vi "rsp_Show Worker Front Panel.vi"(4 "Show in Debugger?":bool=TRUE, 6 "Message Priority":T1=enum."Normal", 8 "error in":errorcluster, 9 "Data in":T2, 11 "Application Manager in":refnum<class "Application Manager.lvclass">) -> (0 "error out":errorcluster, 3 "dup Application Manager out":refnum<class "Application Manager.lvclass">)   [LabVIEW 2017, in "Application Manager.lvclass"]
doc: "This VI sends a <b>Public API Response</b> message to a registered MHL case of the Caller of the Worker that owns this VI.\n---"
uses:
  Application Manager.lvclass
  C:/Program Files (x86)/National Instruments/LabVIEW 2017/vi.lib/addons/_Workers/Library/Classes/Worker/Worker.lvclass
  rsp_Show Worker Front Panel.ctl
  Common VIs/DC_UID.ctl
  <vilib>/addons/_Workers/Library/Classes/Message/Priority.ctl
  Application Manager.lvclass/Application Manager.ctl
  <vilib>/addons/_Workers/Library/Classes/Worker/Worker.lvclass/Worker.ctl
  <vilib>/Utility/error.llb/Error Cluster From Error Code.vi
  <vilib>/ErrorRing/Error Ring.xnode
  <vilib>/addons/_Workers/Library/Classes/Worker/Worker.lvclass
  <vilib>/addons/_Workers/Library/Classes/Message/Message.lvclass
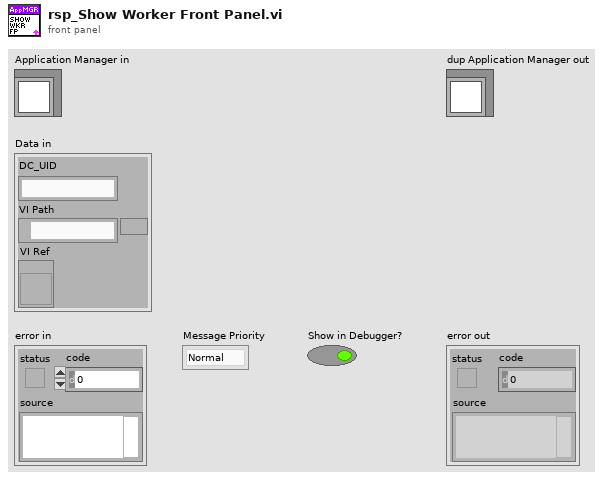
[diagram p1: front panel]
types:
  T1 = typedef "Workers.lvlib/Message.lvclass/Priority.ctl" = enum16{"Low", "Normal", "High"}
  T2 = typedef "Application Manager.lvclass/rsp_Show Worker Front Panel.ctl" = cluster{"DC_UID":T3, "VI Path":path, "VI Ref":refnum<vi>}
  T3 = typedef "DC_UID.ctl" = string
  T4 = typedef "Workers.lvlib/Case Label.ctl" = string
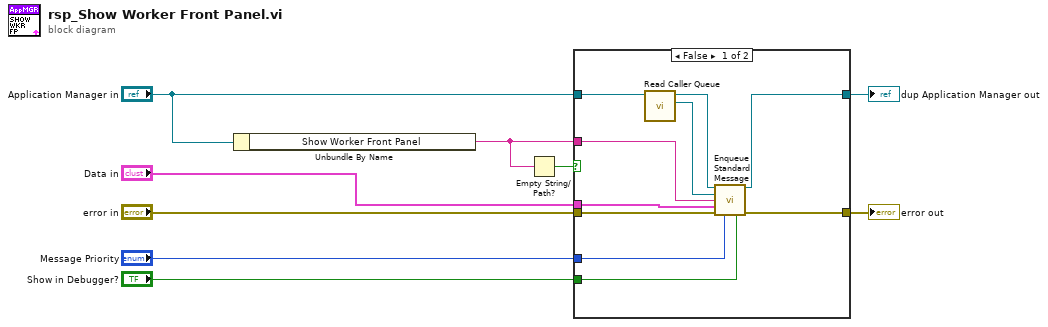
[diagram p0: block diagram]
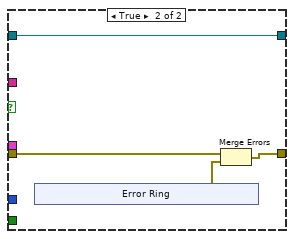
[diagram p2: hidden frame]
diagram:
  n1 = Unbundle By Name("Application Manager in") -> ("Show Worker Front Panel"=w4:T4)
  n2 = Empty String/Path?(string/path=w4) -> (empty?=w5:bool)
  n3 = case shown="False" w5 {
    tunnel: "error in" -> [w16 w20]
    tunnel: [w15 w21] -> w8
    tunnel: "Data in" -> [w12 _]
    tunnel: [w14 w23] -> w6
    tunnel: "Application Manager in" -> [w19 w23]
    tunnel: w4 -> [w13 _]
    tunnel: "Show in Debugger?" -> [w11 _]
    tunnel: "Message Priority" -> [w10 _]
    frame False {
      n4 = call <vilib>:"Read Caller Queue.vi"("Worker_"=w19) -> ("Message Queue out"=w17:refnum<class "Message Queue.lvclass">, "dup Worker_out"=w18:refnum<class "Application Manager.lvclass">)  [unwired: 9 in]
      n5 = call-dynamic "Enqueue Standard Message.vi"("Worker"=w18, "Message Queue"=w17, "Case Label"=w13, "Data"=w12, "error in (no error)"=w16, "Priority (Normal)"=w10, "Send Message to Debugger? (T)"=w11) -> ("dup Worker out"=w14:refnum<class "Application Manager.lvclass">, "error out"=w15:errorcluster)  [unwired: 7 in]
    }
    frame True {
      n6 = xnode "Error Ring"() -> ("error out"=w22:errorcluster)
      n7 = Merge Errors(w20, w22) -> (w21:errorcluster)
    }
  }
  "error out" <- w8
  "dup Application Manager out" <- w6
